vi "ge_GXMLSearchParser.vi"(6 "String ID":string, 8 "error in":errorcluster, 9 "TypeDesc":variant, 10 "XML String In":string) -> (0 "error out":errorcluster, 2 "Parsed Data":variant)   [LabVIEW 2012]
doc: "Using a custom XML schema, this VI converts an XML string into a user specified LabVIEW data type. The data structure is defined by the input <b>TypeDesc</b> and its elements must have the same name and hierarchy as the elements in the XML string.\n\nThis VI employs a recursive searching algorithm so the order of the elements is not important, only their hierarchy. Furthermore since this VI recursively searches for XML content by name, the XML file is allowed to have extra items not referenced by the type definition."
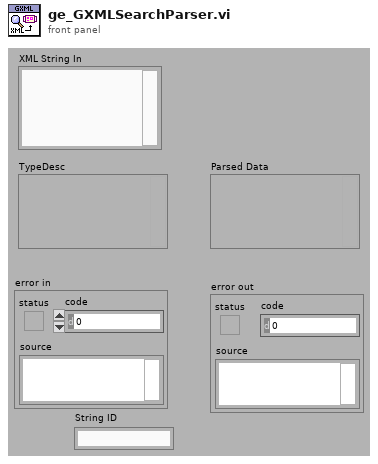
[diagram p1: front panel]
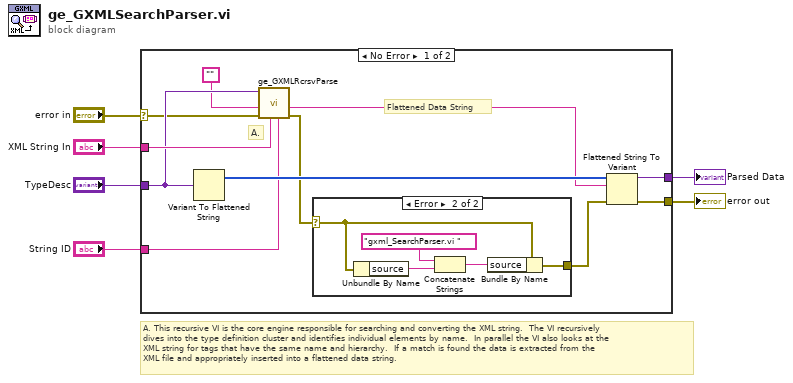
[diagram p0: block diagram]
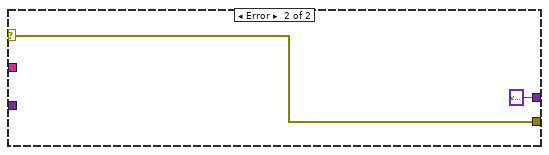
[diagram p3: hidden frame]
diagram:
  # "A. This recursive VI is the core engine responsible for searching and converting the XML string.  The VI recursively \ndives into the type definition cluster and identifies individual elements by name.  In parallel the VI also looks at the \nXML string for tags that have the same name and hierarchy.  If a match is found the data is extracted from the \nXML file and appropriately inserted into a flattened data string."
  n1 = case shown="No Error" "error in" {
    selector: "error in" -> [w9 w25]
    tunnel: [w16 variant ("Variant")] -> w6
    tunnel: "XML String In" -> [w15 _]
    tunnel: "TypeDesc" -> [w14 _]
    tunnel: [w10 w25] -> w3
    tunnel: "String ID" -> [w7 _]
    frame No Error {
      # "Flattened Data String"
      # "A."
      n2 = Variant To Flattened String(Variant=w14) -> (1:w17:i16[])  [unwired: 1 out]
      n3 = call "ge_GXMLRcrsvParse.vi"("String ID"=w7, "File Item Contents"=w15, "error in"=w9, "Flat String In"="", "Item TypeDesc"=w14) -> ("error out"=w12:errorcluster, "Flat String Out"=w13:string)  [unwired: 5 in]
      n4 = case shown="Error" w12 {
        selector: w12 -> [w18 w20]
        tunnel: [w18 w19] -> w11
        frame No Error {
        }
        frame Error {
          n5 = Unbundle By Name(w20) -> ("source"=w23:string)
          n6 = Concatenate Strings("gxml_SearchParser.vi ", w23) -> (w21:string)
          n7 = Bundle By Name(cluster=w20, "source"=w21) -> (w19:errorcluster)
        }
      }
      n8 = Flattened String To Variant(4:w11, 6:w13, 7:w17) -> (0:w10:errorcluster, 3:w16:variant)
    }
    frame Error {
    }
  }
  "error out" <- w3
  "Parsed Data" <- w6
